vi "Establish Connection.vi"(8 "error in (no error)":errorcluster, 11 "Serial_comms in":refnum<class "Serial_comms.lvclass">) -> (0 "error out":errorcluster, 3 "Serial_comms out":refnum<class "Serial_comms.lvclass">)   [LabVIEW 2020, in "Serial_comms.lvlib" / "Serial_comms.lvclass"]
uses:
  Serial_comms.lvclass
  <vilib>/Instr/_visa.llb/VISA Configure Serial Port (Instr).vi
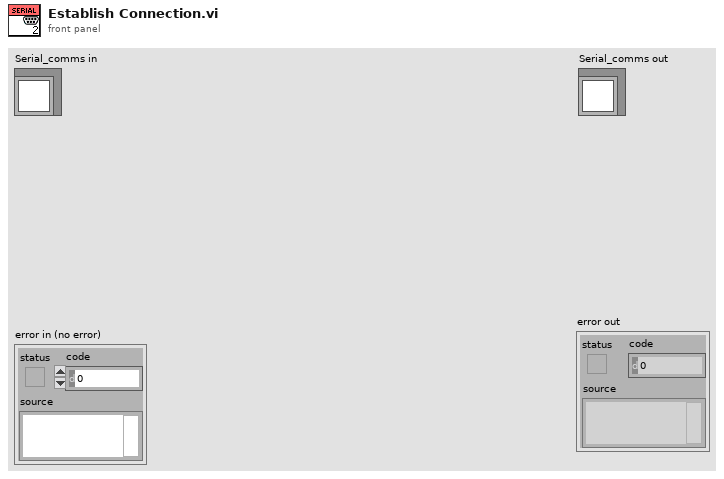
[diagram p1: front panel]
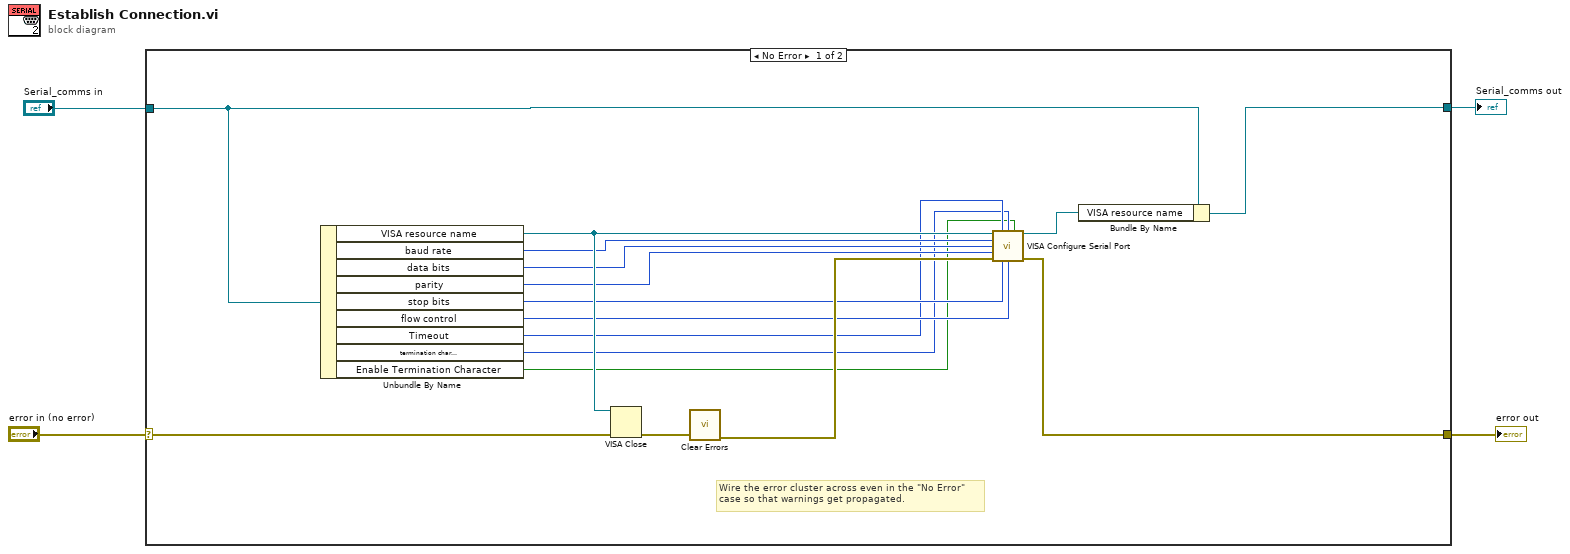
[diagram p0: block diagram]
diagram:
  n1 = case shown="No Error" "error in (no error)" {
    selector: "error in (no error)" -> [w8 w22]
    tunnel: [w7 w22] -> w3
    tunnel: [w5 w21] -> w1
    tunnel: "Serial_comms in" -> [w6 w21]
    frame No Error {
      # "Wire the error cluster across even in the \"No Error\"\ncase so that warnings get propagated."
      n2 = Unbundle By Name(w6) -> ("VISA resource name"=w19:refnum<visa-resource-name>, "baud rate"=w17:u32, "data bits"=w16:u16, "parity"=w15:enum16{"None", "Odd", "Even", "Mark", "Space"}, "stop bits"=w14:u16, "flow control"=w13:u16, "Timeout"=w12:u32, "termination char\n(0xA = '\\n' = LF)"=w11:u8, "Enable Termination Character"=w10:bool)
      n3 = VISA Close(VISA resource name=w19, error in (no error)=w8) -> (error out=w20:errorcluster)
      n4 = call <vilib>:"Clear Errors.vi"("error in (no error)"=w20) -> ("error out"=w18:errorcluster)  [unwired: 5 in, 1 out]
      n5 = call-poly "VISA Configure Serial Port"("VISA resource name"=w19, "timeout (10sec)"=w12, "termination char\n(0xA = '\\n' = LF)"=w11, "Enable Termination\nChar (T)"=w10, "baud rate (9600)"=w17, "data bits (8)"=w16, "parity (0:none)"=w15, "error in (no error)"=w18, "stop bits (10: 1 bit)"=w14, "flow control (0:none)"=w13) -> ("VISA resource name out"=w9:refnum<visa-resource-name>, "error out"=w7:errorcluster)  [unwired: 4 out]
      n6 = Bundle By Name(cluster=w6, "VISA resource name"=w9) -> (w5:refnum<class "Serial_comms.lvclass">)
    }
    frame Error {
    }
  }
  "error out" <- w3
  "Serial_comms out" <- w1
